vi "SogliaLogic.vi"(0 "DSR":refnum<class "DataSocket Tag Reader.lvclass">, 1 "cfg":T1) -> (14 "DSR out":refnum<class "DataSocket Tag Reader.lvclass">, 15 "cfg out":T1, 16 "Array":cluster{bool[], string[]}[](array[cluster]))   [LabVIEW 2018]
uses:
  ControlCfg.ctl
  ControlConfigMisura.ctl
  ControlConfigDI.ctl
  <userlib>/ORI_DataSocketReader/DataSocket Tag Reader.lvclass
  <userlib>/ORI_DataSocketReader/Read Double.vi
  <userlib>/ORI_DataSocketReader/Read Bool.vi
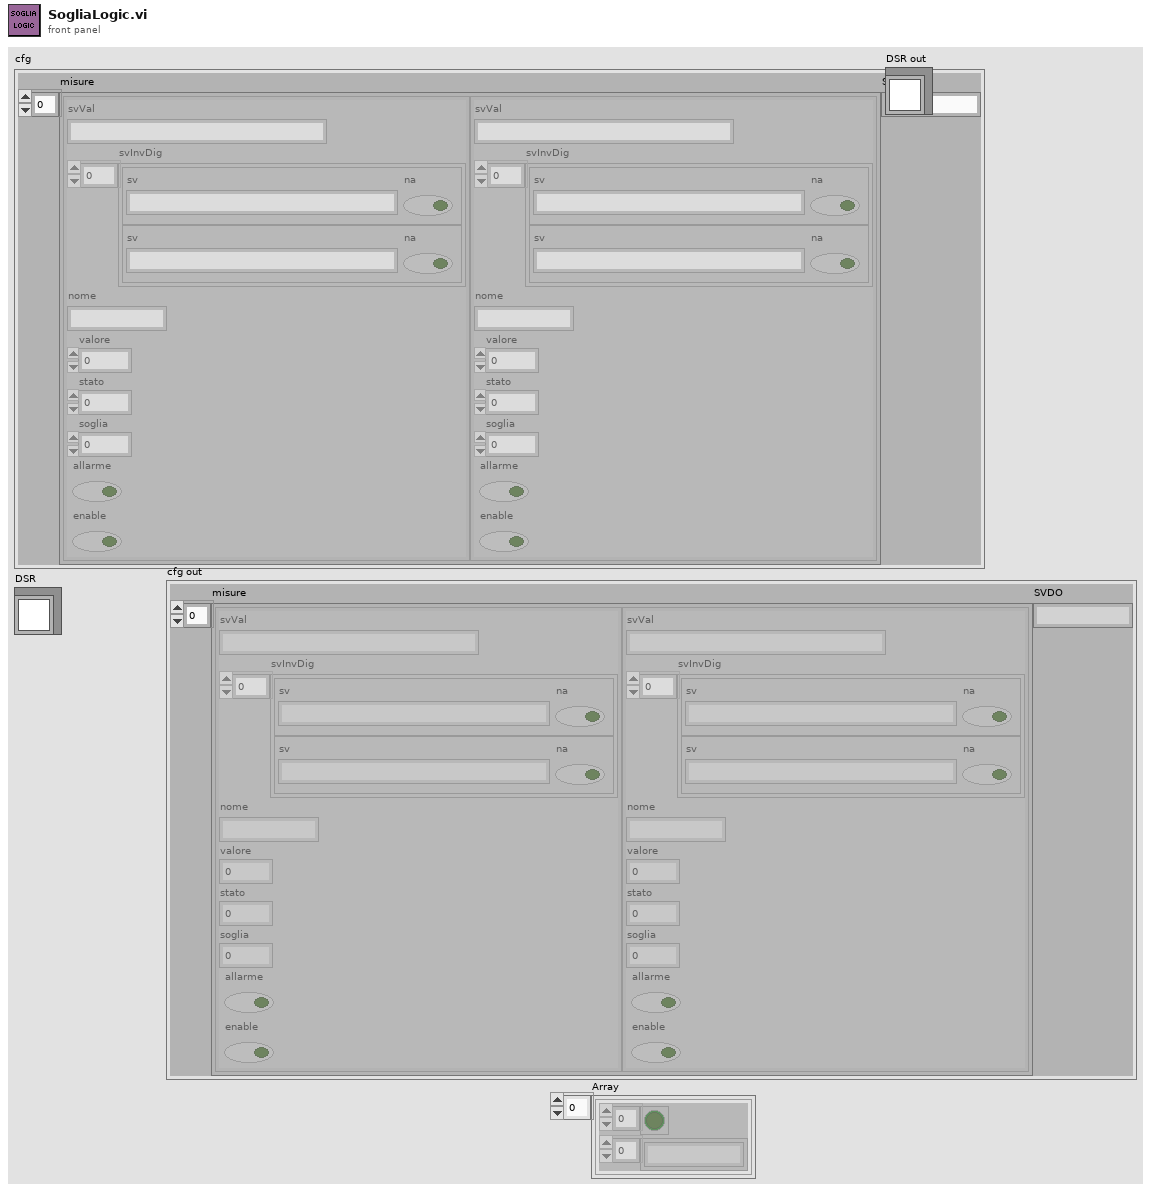
[diagram p1: front panel]
types:
  T1 = typedef "ControlCfg.ctl" = cluster{"misure":T2[], "SVDO":string}
  T2 = typedef "ControlConfigMisura.ctl" = cluster{"svVal":string, "svInvDig":T3[], "nome":string, "valore":dbl, "stato":i16, "soglia":dbl, "allarme":bool, "enable":bool}
  T3 = typedef "ControlConfigDI.ctl" = cluster{"sv":string, "na":bool}
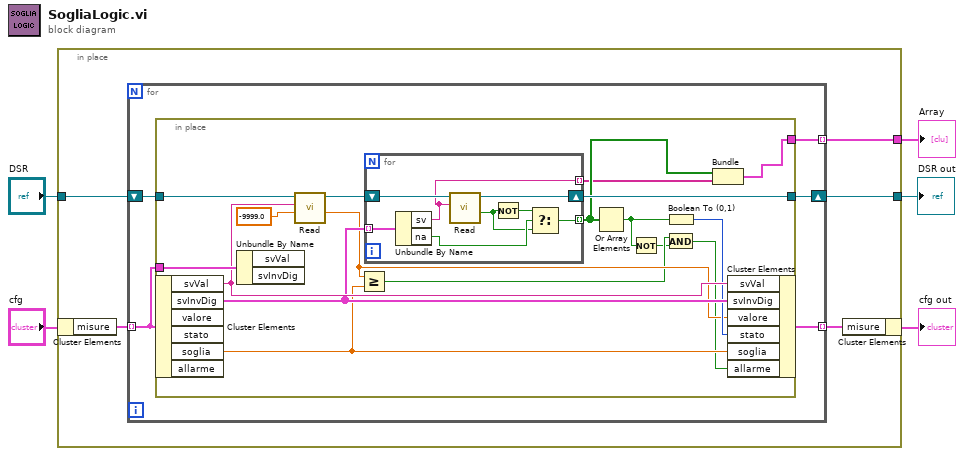
[diagram p0: block diagram]
diagram:
  n1 = in-place {
    in-place-border: "DSR" -> [w10]
    in-place-border: [w7] -> w3
    in-place-border: [w6] -> w1
    n2 = in-place-cluster #1("cfg") -> ("misure"=w9:T2[])
    n3 = for {
      tunnel: w9 -> [w13] mode=indexing
      shift-right: [w14] -> w7
      shift-left: w10 -> [w15]
      tunnel: [w12] -> w8 mode=indexing
      tunnel: [w11] -> w6 mode=indexing
      n4 = in-place {
        in-place-border: w13 -> [w32]
        in-place-border: w15 -> [w31]
        in-place-border: [w29] -> w14
        in-place-border: [w17] -> w11
        n5 = in-place-cluster #2(w13) -> ("svVal"=w28:string, "svInvDig"=w27:T3[], "soglia"=w23:dbl)  [unwired: 3 out]
        n6 = Unbundle By Name(w32) -> ()  [unwired: 2 out]
        n7 = call-poly <userlib>:"Read.vi"("default"=-9999.0, "tag"=w28, "DataSocket Tag Reader in"=w31) -> ("Value"=w24:dbl, "DataSocket Tag Reader out"=w30:refnum<class "DataSocket Tag Reader.lvclass">)  [unwired: 5 in, 2 out]
        n8 = Greater Or Equal?(x=w24, y=w23) -> (x >= y?=w22:bool)
        n9 = for {
          tunnel: w27 -> [w39] mode=indexing
          shift-right: [w38] -> w29
          shift-left: w30 -> [w40]
          tunnel: [w35] -> w18 mode=indexing
          tunnel: [w34] -> w16 mode=indexing
          n10 = Unbundle By Name(w39) -> ("sv"=w34:string, "na"=w37:bool)
          n11 = call-poly <userlib>:"Read.vi"("tag"=w34, "DataSocket Tag Reader in"=w40) -> ("Value"=w33:bool, "DataSocket Tag Reader out"=w38:refnum<class "DataSocket Tag Reader.lvclass">)  [unwired: 6 in, 2 out]
          n12 = Not(x=w33) -> (.not. x?=w36:bool)
          n13 = Select(t=w36, s=w37, f=w33) -> (s? t:f=w35:bool)
        }
        n14 = Or Array Elements(Boolean array=w18) -> (logical OR=w20:bool)
        n15 = Not(x=w20) -> (.not. x?=w21:bool)
        n16 = Boolean To (0,1)(Boolean=w20) -> (0, 1=w25:i16)
        n17 = And(x=w22, y=w21) -> (x .and. y?=w19:bool)
        n18 = Bundle(w18, w16) -> (w17:cluster{bool[], string[]})  [unwired: 1 in]
        n19 = in-place-cluster #2("svVal"=w28, "svInvDig"=w27, "valore"=w24, "stato"=w25, "soglia"=w23, "allarme"=w19) -> (w12:T2)
      }
    }
    n20 = in-place-cluster #1("misure"=w8) -> (→"cfg out":T1)
  }
  "DSR out" <- w3
  "Array" <- w1
